vi "U16 STDEV.vi"(1 "U16 Input Array":u16[](array[numeric])) -> (0 "Standard Deviation":dbl)   [LabVIEW 2013]
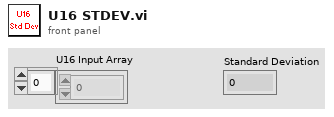
[diagram p1: front panel]
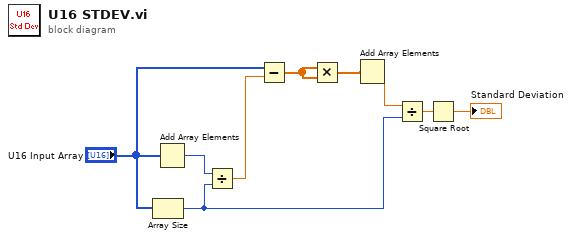
[diagram p0: block diagram]
diagram:
  n1 = Array Size(array="U16 Input Array") -> (size(s)=w3:i32)
  n2 = Add Array Elements(numeric array="U16 Input Array") -> (sum=w8:u16)
  n3 = Divide(x=w8, y=w3) -> (x/y=w7:dbl)
  n4 = Subtract(x="U16 Input Array", y=w7) -> (x-y=w6:dbl[])
  n5 = Multiply(x=w6, y=w6) -> (x*y=w5:dbl[])
  n6 = Add Array Elements(numeric array=w5) -> (sum=w4:dbl)
  n7 = Divide(x=w4, y=w3) -> (x/y=w2:dbl)
  n8 = Square Root(x=w2) -> (sqrt(x)=→"Standard Deviation":dbl)
